vi "Launch Two-Button Dialog Box.vi"(0 "Dialog Launcher In":refnum<class "IViewable.lvclass">, 1 "True Button Return Message (Optional)":refnum<class "Message.lvclass">, 2 "False Button Return Message (Optional)":refnum<class "Message.lvclass">, 3 "Return Priority (Normal)":T1=enum."Normal", 5 "Message Text":string, 7 "True Button Text (OK)":string="OK", 9 "False Button Text (Cancel)":string="Cancel", 11 "error in (no error)":errorcluster, 12 "Modal? (T)":bool=TRUE, 13 "Auto-stop? (T)":bool=TRUE) -> (4 "Dialog Launcher Out":refnum<class "IViewable.lvclass">, 15 "error out":errorcluster)   [LabVIEW 2018, in "MVA Framework.lvlib" / "TwoButtonDialogBox.lvlib" / "TwoButtonDialogBox.lvclass"]
doc: "启动双按钮对话框"
uses:
  TwoButtonDialogBox.lvclass
  IDialogBox/IDialogBox Messages/Dialog Return Msg/Dialog Return Msg.lvclass
  <vilib>/ActorFramework/Actor/Actor.lvclass
  IDialogBox/IDialogBox/IDialogBox.lvclass
  modules/mva-viewable/Source/IViewable/IViewable/IViewable.lvclass
  <vilib>/ActorFramework/Message/Message.lvclass
  <vilib>/ActorFramework/Message Enqueuer/Message Priority.ctl
  <vilib>/ActorFramework/Message Enqueuer/Message Enqueuer.lvclass
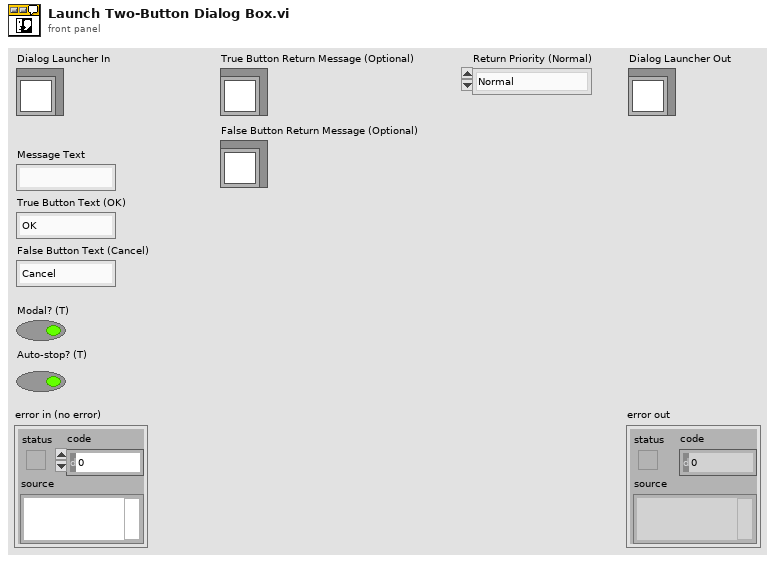
[diagram p1: front panel]
types:
  T1 = typedef "Actor Framework.lvlib/Message Enqueuer.lvclass/Message Priority.ctl" = enum16{"Low", "Normal", "High"}
  T2 = enum32{"Invalid", "Default", "Floating", "Floating/Auto-Hide", "Modal"}
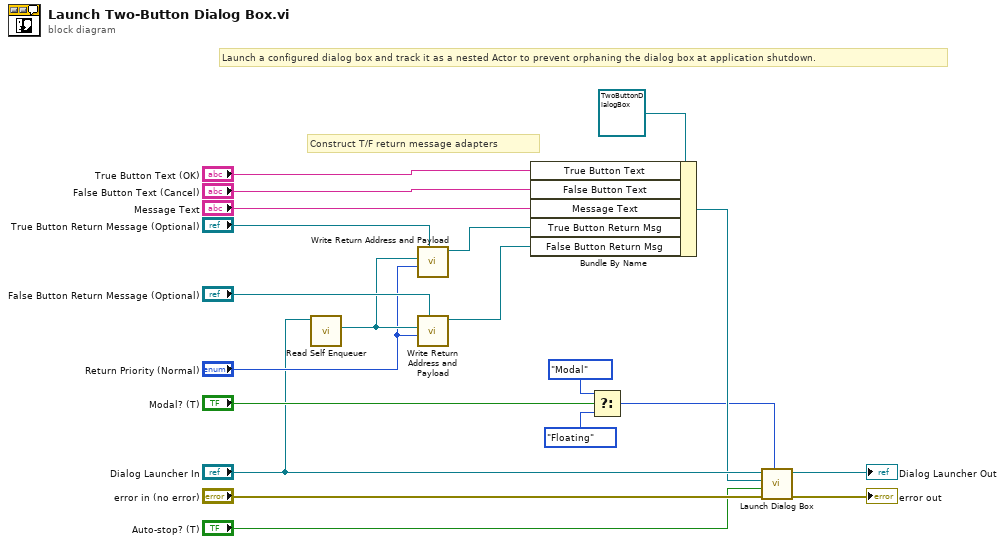
[diagram p0: block diagram]
diagram:
  # "Construct T/F return message adapters"
  # "Launch a configured dialog box and track it as a nested Actor to prevent orphaning the dialog box at application shutdown."
  n1 = call <vilib>:"Read Self Enqueuer.vi"("Actor"="Dialog Launcher In") -> ("Self Enqueuer"=w5:refnum<class "Message Enqueuer.lvclass">)  [unwired: 10 in]
  n2 = call "Write Return Address and Payload.vi"("Reply Message"="True Button Return Message (Optional)", "Return Priority (Normal)"="Return Priority (Normal)", "Return Address"=w5) -> ("Dialog Return Msg out"=w8:refnum<class "Dialog Return Msg.lvclass">)  [unwired: 8 in]
  n3 = call "Write Return Address and Payload.vi"("Reply Message"="False Button Return Message (Optional)", "Return Priority (Normal)"="Return Priority (Normal)", "Return Address"=w5) -> ("Dialog Return Msg out"=w6:refnum<class "Dialog Return Msg.lvclass">)  [unwired: 8 in]
  n4 = Bundle By Name(cluster=refnum<class "TwoButtonDialogBox.lvclass"> refnum ("OneButtonDialogBox in"), "True Button Text"="True Button Text (OK)", "False Button Text"="False Button Text (Cancel)", "Message Text"="Message Text", "True Button Return Msg"=w8, "False Button Return Msg"=w6) -> (w2:refnum<class "TwoButtonDialogBox.lvclass">)
  n5 = Select(t=T2."Modal" ("FP Window:Behavior"), s="Modal? (T)", f=T2."Floating" ("FP Window:Behavior")) -> (s? t:f=w1:T2)
  n6 = call "Launch Dialog Box.vi"("FP Window:Behavior (Floating)"=w1, "error in (no error)"="error in (no error)", "Auto-stop? (T)"="Auto-stop? (T)", "DialogBox"=w2, "DialogBox Launcher"="Dialog Launcher In") -> ("error out"=→"error out":errorcluster, "DialogBox Launcher Out"=→"Dialog Launcher Out":refnum<class "IViewable.lvclass">)  [unwired: 4 in, 1 out]
